vi "SMO.UI.ErrorTester.GetPublicEvents.vi"(8 "error in (no error)":errorcluster, 11 "SMO.UI.ByRefWithEvents":refnum<class "SMO.UI.ErrorTester.lvclass">) -> (0 "error out":errorcluster, 2 "SMO.Template Public Events":T1, 3 "SMO.UI.ByRefWithEvents out":refnum<class "SMO.UI.ErrorTester.lvclass">)   [LabVIEW 2013, in "SMO.UI.ErrorTester.lvclass"]
doc: "---------------------------------------------------------------\nJKI State Machine Objects™\nhttp://jki.net/state-machine-objects/\nCopyright (C) 2005-2015, JKI <info@jki.net>\nALL RIGHTS RESERVEDJKI State Machine Objects (SMO) 1.0.0.5\nJKI - JKI\nCopyright (c) 2016, JKI"
uses:
  SMO.UI.ErrorTester.lvclass
  Typedefs/PublicEvents--Cluster.ctl
  Typedefs/DataChanged--EventData--Cluster.ctl
  SMO.UI.ErrorTester.lvclass/SMO.UI.ErrorTester.ctl
panel:
  # "For instructions on how to use the JKI State Machine Objects, examples and video tutorials, visit:\nhttp://jki.net/state-machine-objects/\n\nJKI State Machine Objects™\nhttp://jki.net/state-machine-objects/\nCopyright (C) 2005-2015, JKI <info@jki.net>\nALL RIGHTS RESERVED"
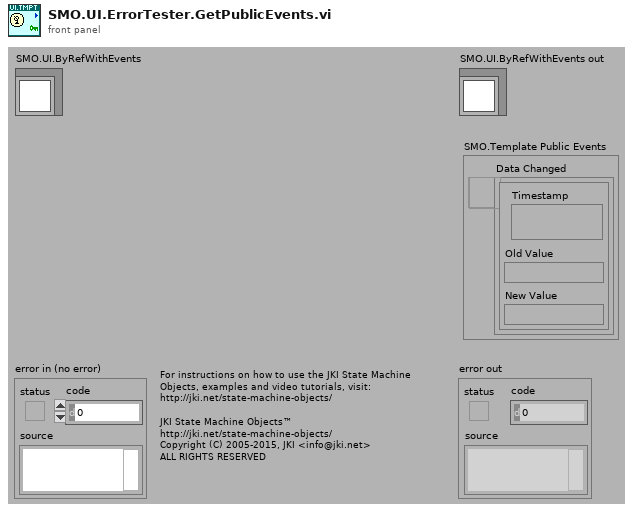
[diagram p1: front panel]
types:
  T1 = typedef "SMO.UI.ErrorTester.lvclass/PublicEvents--Cluster.ctl" = cluster{"Data Changed":refnum<user-event>}
  T2 = typedef "SMO.UI.ErrorTester.lvclass/PrivateData--Ref.ctl" = refnum<data-value>
  T3 = typedef "SMO.UI.ErrorTester.lvclass/PrivateData--Cluster.ctl" = cluster{"Configuration":T4, "Public Events":T1, "Protected Events":T5, "Data":string}
  T4 = typedef "SMO.UI.ErrorTester.lvclass/Configuration--Cluster.ctl" = cluster{"Suffix":string}
  T5 = typedef "SMO.UI.ErrorTester.lvclass/ProtectedEvents--Cluster.ctl" = cluster{"ErrorGeneration":refnum<user-event>}
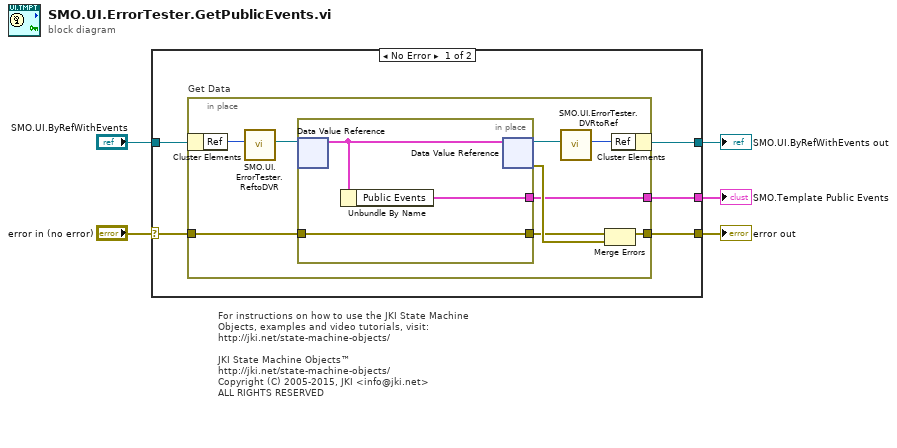
[diagram p0: block diagram]
diagram:
  # "For instructions on how to use the JKI State Machine Objects, examples and video tutorials, visit:\nhttp://jki.net/state-machine-objects/\n\nJKI State Machine Objects™\nhttp://jki.net/state-machine-objects/\nCopyright (C) 2005-2015, JKI <info@jki.net>\nALL RIGHTS RESERVED"
  n1 = case shown="No Error" "error in (no error)" {
    selector: "error in (no error)" -> [w9 w23]
    tunnel: "SMO.UI.ByRefWithEvents" -> [w10 w24]
    tunnel: [w8 w23] -> w4
    tunnel: [w7 w24] -> w3
    tunnel: [w6 _] -> w1
    frame No Error {
      n2 = in-place "Get Data" {
        in-place-border: w9 -> [w19]
        in-place-border: [w16] -> w8
        in-place-border: [w15] -> w6
        n3 = in-place-cluster #1(w10) -> ("Ref"=w14:u32)
        n4 = call "SMO.UI.ErrorTester.ReftoDVR.vi"("Ref"=w14) -> ("Ref"=w13:T2)  [unwired: 10 in]
        n5 = in-place {
          in-place-border: w19 -> [w21]
          in-place-border: [w21] -> w17
          in-place-border: [w20] -> w15
          n6 = in-place-dvr #2(w13) -> (w22:T3)  [unwired: 1 out]
          n7 = Unbundle By Name(w22) -> ("Public Events"=w20:T1)
          n8 = in-place-dvr #2(w22) -> (w12:T2, w18:errorcluster)
        }
        n9 = call "SMO.UI.ErrorTester.DVRtoRef.vi"("Ref"=w12) -> ("Ref"=w11:u32)  [unwired: 10 in]
        n10 = Merge Errors(w17, w18) -> (w16:errorcluster)
        n11 = in-place-cluster #1("Ref"=w11) -> (w7:refnum<class "SMO.UI.ErrorTester.lvclass">)
      }
    }
    frame Error {
    }
  }
  "error out" <- w4
  "SMO.UI.ByRefWithEvents out" <- w3
  "SMO.Template Public Events" <- w1
